vi "Untitled 1.vi"() -> ()   [LabVIEW 2015]
uses:
  <instrlib>/_niInstr/Basic Elements/v1/FPGA/Private/Count Up U64.vi
  <instrlib>/_niInstr/Basic Elements/v1/FPGA/niInstr Basic Elements v1 FPGA.lvlib
panel:
  in  "set":bool
  out "out":bool
  in  "trigger \ndelay":u64
  in  "Clear Trigger":bool
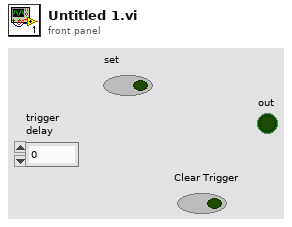
[diagram p1: front panel]
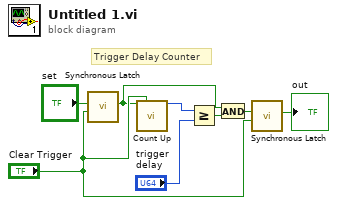
[diagram p0: block diagram]
diagram:
  # "Trigger Delay Counter"
  n1 = call <instrlib>:"Synchronous Latch.vi"("clear"="Clear Trigger", "set"="set") -> ("out"=w4:bool)  [unwired: 9 in]
  n2 = call-poly <instrlib>:"Count Up.vi"("increment"=w4, "reset"="Clear Trigger") -> ("count out"=w8:u64)  [unwired: 13 in]
  n3 = Greater Or Equal?(x=w8, y="trigger \ndelay") -> (x >= y?=w5:bool)
  n4 = And(x=w4, y=w5) -> (x .and. y?=w3:bool)
  n5 = call <instrlib>:"Synchronous Latch.vi"("clear"="Clear Trigger", "set"=w3) -> ("out"=→"out":bool)  [unwired: 9 in]
